vi "Teleop.vi"(10 "Match Info":T1={"Autonomous Elapsed Seconds"=0.0, "TeleOp Elapsed Seconds"=0.0, "Disabled Elapsed Seconds"=0.0, "Visited Autonomous"=FALSE, "Visited TeleOp"=FALSE, "Visited Disabled"=FALSE, "Autonomous Settings"={"Autonomous Style"=enum."Independent", "VI Refnum"=refnum}}, 11 "Call Context":T2) -> ()   [LabVIEW 2016]
doc: "This VI is called for each TeleOp packet received from the DS where the robot is not disabled. It is often used to read from the joysticks and update I/O or to update setpoints for timed control loops. It should complete and return within 20 milliseconds or it may miss DS packets."
uses:
  <vilib>/Rock Robotics/WPI/DriverStation/WPI_DriverStationDerivedRobotMode.ctl
  <vilib>/Rock Robotics/WPI/DriverStation/WPI_DriverStationMatch Info.ctl
  <vilib>/Rock Robotics/WPI/Solenoid/WPI_SolenoidValue.ctl
  <vilib>/Rock Robotics/Network Tables/NT Read Boolean.vi
  <vilib>/Rock Robotics/Network Tables/NT Read Number.vi
  <vilib>/Rock Robotics/WPI/Utilities/WPI_GetSetVariantRefNum.vi
  <vilib>/Rock Robotics/WPI/Solenoid/Deprecated/WPI_SolenoidSetBool.vi
  <vilib>/Rock Robotics/Network Tables/NT Write Number.vi
  <vilib>/Rock Robotics/WPI/Solenoid/WPI_SolenoidSetEnum.vi
panel:
  out "Distance 2":dbl
  out "Distance":dbl
  out "Sample Slider 0":dbl(slide) scale=0.0..5.0
  out "Sample Boolean 1":bool
  out "Sample Boolean 0":bool
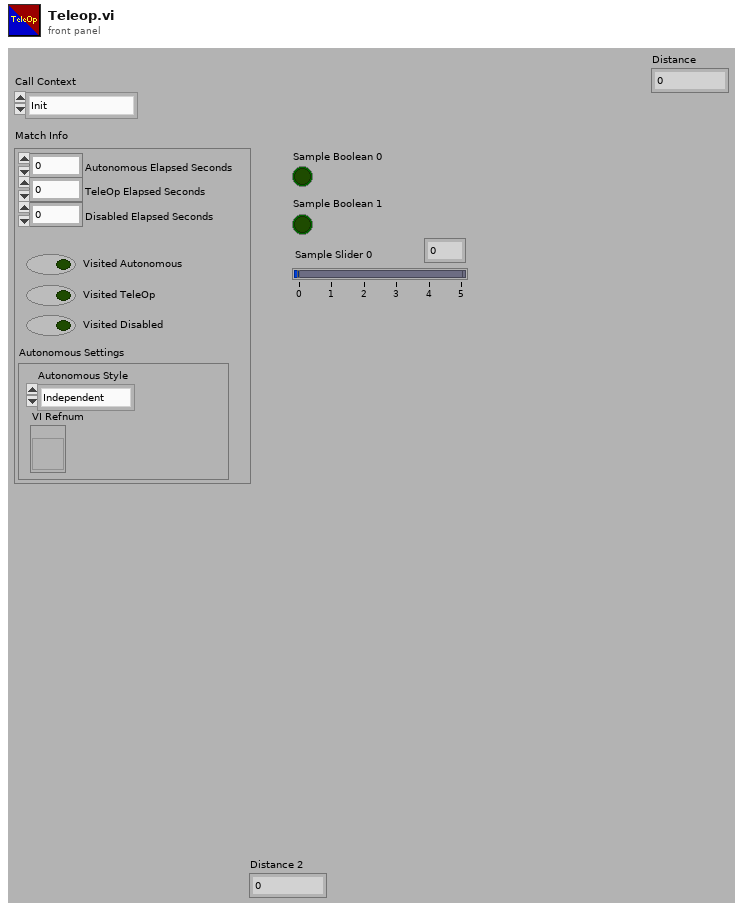
[diagram p1: front panel]
types:
  T1 = typedef "WPI_DriverStationMatch Info.ctl" = cluster{"Autonomous Elapsed Seconds":dbl, "TeleOp Elapsed Seconds":dbl, "Disabled Elapsed Seconds":dbl, "Visited Autonomous":bool, "Visited TeleOp":bool, "Visited Disabled":bool, "Autonomous Settings":cluster{"Autonomous Style":enum16{"Iterative", "Independent"}, "VI Refnum":refnum<vi>}}
  T2 = typedef "WPI_DriverStationDerivedRobotMode.ctl" = enum16{"Init", "Execute", "Stop"}
  T3 = typedef "WPI_JoystickDevRef.ctl" = cluster{"Device":T4}
  T4 = typedef "WPI_JoystickDeviceEnum.ctl" = enum16{"USB 0", "USB 1", "USB 2", "USB 3", "USB 4", "USB 5"}
  T5 = typedef "WPI_EncoderDevRef.ctl" = cluster{"DevStatus":errorcluster, "EncoderIndex":T6, "CounterIndex":T7, "DistancePerCount":dbl, "Decoding Type":T8}
  T6 = typedef "FPGA_EncoderIdx.ctl" = enum8{"Enc 0", "Enc 1", "Enc 2", "Enc 3", "Enc 4", "Enc 5", "Enc 6", "Enc 7", "Invalid"}
  T7 = typedef "FPGA_CounterCtrSystemIndex.ctl" = enum8{"Ctr 0", "Ctr 1", "Ctr 2", "Ctr 3", "Ctr 4", "Ctr 5", "Ctr 6", "Ctr 7", "Invalid"}
  T8 = typedef "WPI_EncoderType.ctl" = enum16{"1x", "2x", "4x"}
  T9 = typedef "WPI_MotorControlDeviceRef.ctl" = cluster{"DeviceStatus":errorcluster, "Type":T10, "PWM":cluster{"PWM Channel":T11, "DeadBand":T12}, "CAN":cluster{"Device Number":u8, "SetOutput VI Ref":variant, "GetOutput VI Ref":variant, "Enable VI Ref":variant, "Disable VI Ref":variant, "Data":variant}, "Invert":bool}
  T10 = typedef "WPI_MotorControlType.ctl" = enum16{"PWM", "CAN"}
  T11 = typedef "FPGA_DIOPWMChannel.ctl" = enum8{"PWM 0", "PWM 1", "PWM 2", "PWM 3", "PWM 4", "PWM 5", "PWM 6", "PWM 7", "PWM 8", "PWM 9", "PWM MXP 0", "PWM MXP 1", "PWM MXP 2", "PWM MXP 3", "PWM MXP 4", "PWM MXP 5", "PWM MXP 6", "PWM MXP 7", "PWM MXP 8", "PWM MXP 9", "Invalid"}
  T12 = typedef "WPI_PWMDeadband.ctl" = cluster{"Name":string, "maxPositivePwm":i32, "minPositivePwm":i32, "centerPwm":i32, "maxNegativePwm":i32, "minNegativePwm":i32, "angularRange":u16}
  T13 = typedef "WPI_RobotDriveDevRef.ctl" = cluster{"DevStatus":errorcluster, "Motors[]":T9[], "Square Inputs":bool, "Max Output":dbl}
  T14 = typedef "WPI_CompressorDevRef.ctl" = cluster{"DevStatus":errorcluster, "Pneumatics Control Module":u8}
  T15 = typedef "WPI_SolenoidValue.ctl" = enum16{"Off", "On", "Forward", "Reverse"}
  T16 = typedef "WPI_SolenoidDevRef.ctl" = cluster{"DevStatus":errorcluster, "Pneumatics Control Module":u8, "Forward Solenoid Channel":T17, "Reverse Solenoid Channel":T17}
  T17 = typedef "WPI_SolenoidChannel.ctl" = enum8{"Solenoid 0", "Solenoid 1", "Solenoid 2", "Solenoid 3", "Solenoid 4", "Solenoid 5", "Solenoid 6", "Solenoid 7", "Invalid"}
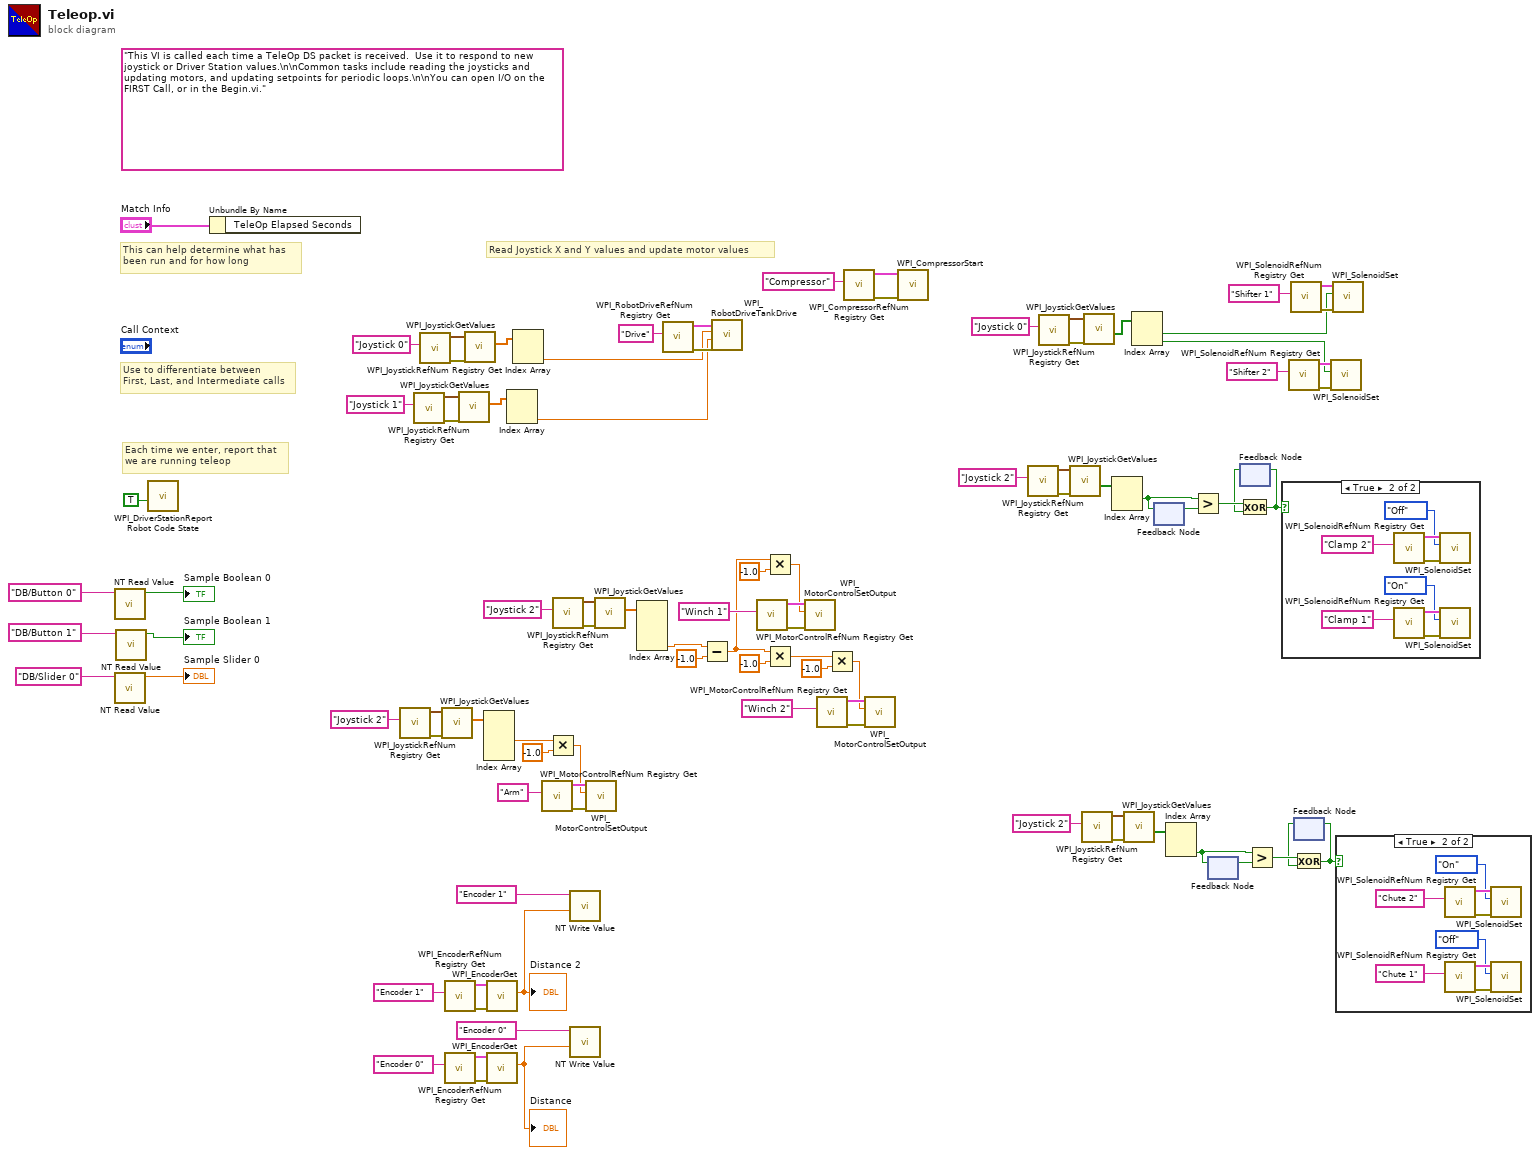
[diagram p0: block diagram]
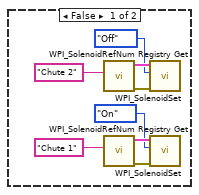
[diagram p2: hidden frame]
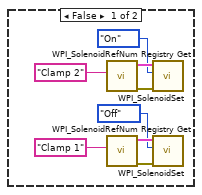
[diagram p3: hidden frame]
diagram:
  (unwired) "This VI is called each time a TeleOp DS packet is received.  Use it to respond to new joystick or Driver Station values.\n\nCommon tasks include reading the joysticks and updating motors, and updating setpoints for periodic loops.\n\nYou can open I/O on the FIRST Call, or in the Begin.vi."
  # "Each time we enter, report that\nwe are running teleop"
  # "Use to differentiate between\nFirst, Last, and Intermediate calls"
  # "This can help determine what has\nbeen run and for how long"
  # "Read Joystick X and Y values and update motor values"
  n1 = call-poly <vilib>:"NT Read Value.vi"("Name"="DB/Button 0" ("refnum name")) -> ("Boolean"=→"Sample Boolean 0":bool)  [unwired: 9 in, 1 out]
  n2 = call-poly <vilib>:"NT Read Value.vi"("Name"="DB/Slider 0" ("refnum name")) -> ("Numeric"=→"Sample Slider 0":dbl)  [unwired: 9 in, 1 out]
  n3 = call-poly <vilib>:"NT Read Value.vi"("Name"="DB/Button 1" ("refnum name")) -> ("Boolean"=→"Sample Boolean 1":bool)  [unwired: 9 in, 1 out]
  n4 = call <vilib>:"WPI_DriverStationReport Robot Code State.vi"("TeleOp"=TRUE ("Autonomous")) -> ()  [unwired: 10 in, 1 out]
  n5 = Unbundle By Name("Match Info") -> ()  [unwired: 1 out]
  n6 = call <vilib>:"WPI_JoystickRefNum Registry Get.vi"("refnum name"="Joystick 2") -> ("error out"=w41:errorcluster, "JoystickDevRef"=w40:T3)  [unwired: 9 in]
  n7 = call <vilib>:"WPI_JoystickRefNum Registry Get.vi"("refnum name"="Joystick 1") -> ("error out"=w81:errorcluster, "JoystickDevRef"=w80:T3)  [unwired: 9 in]
  n8 = call <vilib>:"WPI_JoystickRefNum Registry Get.vi"("refnum name"="Joystick 0") -> ("error out"=w85:errorcluster, "JoystickDevRef"=w84:T3)  [unwired: 9 in]
  n9 = call <vilib>:"WPI_JoystickGetValues.vi"("error in (no error)"=w41, "JoystickDevRef"=w40) -> ("Axes"=w38:dbl[])  [unwired: 5 in, 4 out]
  n10 = call <vilib>:"WPI_EncoderRefNum Registry Get.vi"("refnum name"="Encoder 1") -> ("error out"=w7:errorcluster, "EncoderDevRef"=w6:T5)  [unwired: 9 in]
  n11 = call <vilib>:"WPI_EncoderRefNum Registry Get.vi"("refnum name"="Encoder 0") -> ("error out"=w10:errorcluster, "EncoderDevRef"=w9:T5)  [unwired: 9 in]
  n12 = call <vilib>:"WPI_JoystickGetValues.vi"("error in (no error)"=w81, "JoystickDevRef"=w80) -> ("Axes"=w78:dbl[])  [unwired: 5 in, 4 out]
  n13 = call <vilib>:"WPI_JoystickGetValues.vi"("error in (no error)"=w85, "JoystickDevRef"=w84) -> ("Axes"=w82:dbl[])  [unwired: 5 in, 4 out]
  n14 = Index Array(array=w38) -> (element #2=w37:dbl)  [unwired: 4 in, 3 out]
  n15 = call <vilib>:"WPI_EncoderGet.vi"("error in (no error)"=w7, "EncoderDevRef"=w6) -> ("Distance"=w2:dbl)  [unwired: 4 in, 5 out]
  "Distance 2" <- w2
  n16 = call <vilib>:"WPI_EncoderGet.vi"("error in (no error)"=w10, "EncoderDevRef"=w9) -> ("Distance"=w4:dbl)  [unwired: 4 in, 5 out]
  "Distance" <- w4
  n17 = Index Array(array=w78) -> (element #2=w73:dbl)  [unwired: 2 in, 1 out]
  n18 = Index Array(array=w82) -> (element #2=w74:dbl)  [unwired: 2 in, 1 out]
  n19 = call <vilib>:"WPI_MotorControlRefNum Registry Get.vi"("refnum name"="Arm") -> ("error out"=w34:errorcluster, "MotorControlDevRef"=w35:T9)  [unwired: 9 in]
  n20 = Multiply(x=w37, y=-1.0) -> (x*y=w32:dbl)
  n21 = call <vilib>:"WPI_JoystickRefNum Registry Get.vi"("refnum name"="Joystick 2") -> ("error out"=w72:errorcluster, "JoystickDevRef"=w71:T3)  [unwired: 9 in]
  n22 = call-poly <vilib>:"NT Write Value.vi"("Numeric"=w2, "Name"="Encoder 1") -> ()  [unwired: 9 in, 1 out]
  n23 = call-poly <vilib>:"NT Write Value.vi"("Numeric"=w4, "Name"="Encoder 0") -> ()  [unwired: 9 in, 1 out]
  n24 = call <vilib>:"WPI_MotorControlSetOutput.vi"("error in (no error)"=w34, "Output"=w32, "MotorControlDevRef"=w35) -> ()  [unwired: 6 in, 3 out]
  n25 = call <vilib>:"WPI_JoystickGetValues.vi"("error in (no error)"=w72, "JoystickDevRef"=w71) -> ("Axes"=w69:dbl[])  [unwired: 5 in, 4 out]
  n26 = Index Array(array=w69) -> (element #4=w61:dbl)  [unwired: 4 in, 3 out]
  n27 = call <vilib>:"WPI_RobotDriveRefNum Registry Get.vi"("refnum name"="Drive") -> ("error out"=w76:errorcluster, "RobotDriveDevRef"=w77:T13)  [unwired: 9 in]
  n28 = Subtract(x=w61, y=-1.0) -> (x-y=w57:dbl)
  n29 = call <vilib>:"WPI_RobotDriveTankDrive.vi"("error in (no error)"=w76, "Right axis value"=w73, "Left axis value"=w74, "RobotDriveDevRef"=w77) -> ()  [unwired: 5 in, 3 out]
  n30 = call <vilib>:"WPI_MotorControlRefNum Registry Get.vi"("refnum name"="Winch 1") -> ("error out"=w68:errorcluster, "MotorControlDevRef"=w67:T9)  [unwired: 9 in]
  n31 = Multiply(x=w57, y=-1.0) -> (x*y=w58:dbl)
  n32 = Multiply(x=w57, y=-1.0) -> (x*y=w42:dbl)
  n33 = call <vilib>:"WPI_MotorControlSetOutput.vi"("error in (no error)"=w68, "Output"=w58, "MotorControlDevRef"=w67) -> ()  [unwired: 6 in, 3 out]
  n34 = call <vilib>:"WPI_MotorControlRefNum Registry Get.vi"("refnum name"="Winch 2") -> ("error out"=w65:errorcluster, "MotorControlDevRef"=w64:T9)  [unwired: 9 in]
  n35 = Multiply(x=w42, y=-1.0) -> (x*y=w43:dbl)
  n36 = call <vilib>:"WPI_CompressorRefNum Registry Get.vi"("refnum name"="Compressor") -> ("error out"=w46:errorcluster, "CompressorDevRef"=w47:T14)  [unwired: 9 in]
  n37 = call <vilib>:"WPI_MotorControlSetOutput.vi"("error in (no error)"=w65, "Output"=w43, "MotorControlDevRef"=w64) -> ()  [unwired: 6 in, 3 out]
  n38 = call <vilib>:"WPI_CompressorStart.vi"("error in (no error)"=w46, "CompressorDevRef"=w47) -> ()  [unwired: 8 in, 2 out]
  n39 = call <vilib>:"WPI_JoystickRefNum Registry Get.vi"("refnum name"="Joystick 2") -> ("error out"=w56:errorcluster, "JoystickDevRef"=w55:T3)  [unwired: 9 in]
  n40 = call <vilib>:"WPI_JoystickRefNum Registry Get.vi"("refnum name"="Joystick 0") -> ("error out"=w31:errorcluster, "JoystickDevRef"=w30:T3)  [unwired: 9 in]
  n41 = call <vilib>:"WPI_JoystickGetValues.vi"("error in (no error)"=w56, "JoystickDevRef"=w55) -> ("Buttons"=w53:bool[])  [unwired: 5 in, 4 out]
  n42 = call <vilib>:"WPI_JoystickRefNum Registry Get.vi"("refnum name"="Joystick 2") -> ("error out"=w19:errorcluster, "JoystickDevRef"=w18:T3)  [unwired: 9 in]
  n43 = call <vilib>:"WPI_JoystickGetValues.vi"("error in (no error)"=w31, "JoystickDevRef"=w30) -> ("Buttons"=w28:bool[])  [unwired: 5 in, 4 out]
  n44 = Index Array(array=w53) -> (element #1=w51:bool)  [unwired: 2 in, 1 out]
  n45 = call <vilib>:"WPI_JoystickGetValues.vi"("error in (no error)"=w19, "JoystickDevRef"=w18) -> ("Buttons"=w16:bool[])  [unwired: 5 in, 4 out]
  n46 = Index Array(array=w28) -> (element #1=w21:bool, element #2=w20:bool)  [unwired: 2 in]
  n47 = feedback #1() -> (w52:bool)  [unwired: 1 in]
  n48 = feedback-in #1(w51) -> ()
  n49 = Index Array(array=w16) -> (element #2=w11:bool)  [unwired: 2 in, 1 out]
  n50 = Greater?(x=w51, y=w52) -> (0:w50:bool)
  n51 = feedback #2() -> (w15:bool)  [unwired: 1 in]
  n52 = feedback-in #2(w11) -> ()
  n53 = feedback #3() -> (w49:bool)  [unwired: 1 in]
  n54 = Exclusive Or(1:w49, 2:w50) -> (0:w48:bool)
  n55 = feedback-in #3(w48) -> ()
  n56 = Greater?(x=w11, y=w15) -> (0:w14:bool)
  n57 = case shown="True" w48 {
    frame False {
      n58 = call <vilib>:"WPI_SolenoidRefNum Registry Get.vi"("refnum name"="Clamp 2") -> ("error out"=w101:errorcluster, "SolenoidDevRef"=w100:T16)  [unwired: 9 in]
      n59 = call <vilib>:"WPI_SolenoidRefNum Registry Get.vi"("refnum name"="Clamp 1") -> ("error out"=w98:errorcluster, "SolenoidDevRef"=w97:T16)  [unwired: 9 in]
      n60 = call-poly <vilib>:"WPI_SolenoidSet.vi"("error in (no error)"=w101, "Value"=WPI_SolenoidValue."On", "SolenoidDevRef"=w100) -> ()  [unwired: 7 in, 2 out]
      n61 = call-poly <vilib>:"WPI_SolenoidSet.vi"("error in (no error)"=w98, "Value"=WPI_SolenoidValue."Off", "SolenoidDevRef"=w97) -> ()  [unwired: 7 in, 2 out]
    }
    frame True {
      n62 = call <vilib>:"WPI_SolenoidRefNum Registry Get.vi"("refnum name"="Clamp 2") -> ("error out"=w109:errorcluster, "SolenoidDevRef"=w108:T16)  [unwired: 9 in]
      n63 = call <vilib>:"WPI_SolenoidRefNum Registry Get.vi"("refnum name"="Clamp 1") -> ("error out"=w106:errorcluster, "SolenoidDevRef"=w105:T16)  [unwired: 9 in]
      n64 = call-poly <vilib>:"WPI_SolenoidSet.vi"("error in (no error)"=w109, "Value"=WPI_SolenoidValue."Off", "SolenoidDevRef"=w108) -> ()  [unwired: 7 in, 2 out]
      n65 = call-poly <vilib>:"WPI_SolenoidSet.vi"("error in (no error)"=w106, "Value"=WPI_SolenoidValue."On", "SolenoidDevRef"=w105) -> ()  [unwired: 7 in, 2 out]
    }
  }
  n66 = call <vilib>:"WPI_SolenoidRefNum Registry Get.vi"("refnum name"="Shifter 2") -> ("error out"=w24:errorcluster, "SolenoidDevRef"=w23:T16)  [unwired: 9 in]
  n67 = call <vilib>:"WPI_SolenoidRefNum Registry Get.vi"("refnum name"="Shifter 1") -> ("error out"=w27:errorcluster, "SolenoidDevRef"=w26:T16)  [unwired: 9 in]
  n68 = feedback #4() -> (w12:bool)  [unwired: 1 in]
  n69 = Exclusive Or(1:w12, 2:w14) -> (0:w13:bool)
  n70 = feedback-in #4(w13) -> ()
  n71 = call-poly <vilib>:"WPI_SolenoidSet.vi"("error in (no error)"=w24, "Value"=w20, "SolenoidDevRef"=w23) -> ()  [unwired: 7 in, 2 out]
  n72 = call-poly <vilib>:"WPI_SolenoidSet.vi"("error in (no error)"=w27, "Value"=w21, "SolenoidDevRef"=w26) -> ()  [unwired: 7 in, 2 out]
  n73 = case shown="True" w13 {
    frame False {
      n74 = call <vilib>:"WPI_SolenoidRefNum Registry Get.vi"("refnum name"="Chute 2") -> ("error out"=w117:errorcluster, "SolenoidDevRef"=w116:T16)  [unwired: 9 in]
      n75 = call <vilib>:"WPI_SolenoidRefNum Registry Get.vi"("refnum name"="Chute 1") -> ("error out"=w114:errorcluster, "SolenoidDevRef"=w113:T16)  [unwired: 9 in]
      n76 = call-poly <vilib>:"WPI_SolenoidSet.vi"("error in (no error)"=w117, "Value"=WPI_SolenoidValue."Off", "SolenoidDevRef"=w116) -> ()  [unwired: 7 in, 2 out]
      n77 = call-poly <vilib>:"WPI_SolenoidSet.vi"("error in (no error)"=w114, "Value"=WPI_SolenoidValue."On", "SolenoidDevRef"=w113) -> ()  [unwired: 7 in, 2 out]
    }
    frame True {
      n78 = call <vilib>:"WPI_SolenoidRefNum Registry Get.vi"("refnum name"="Chute 2") -> ("error out"=w125:errorcluster, "SolenoidDevRef"=w124:T16)  [unwired: 9 in]
      n79 = call <vilib>:"WPI_SolenoidRefNum Registry Get.vi"("refnum name"="Chute 1") -> ("error out"=w122:errorcluster, "SolenoidDevRef"=w121:T16)  [unwired: 9 in]
      n80 = call-poly <vilib>:"WPI_SolenoidSet.vi"("error in (no error)"=w125, "Value"=WPI_SolenoidValue."On", "SolenoidDevRef"=w124) -> ()  [unwired: 7 in, 2 out]
      n81 = call-poly <vilib>:"WPI_SolenoidSet.vi"("error in (no error)"=w122, "Value"=WPI_SolenoidValue."Off", "SolenoidDevRef"=w121) -> ()  [unwired: 7 in, 2 out]
    }
  }
